vi "Configure Channel Probe.vi"(6 "Probe Signal Type (1: Single-ended)":i32(ring)=1 items=["Differential", "Single-ended"], 7 "Skew Factor (1E-7 S)":dbl=1e-07, 8 "error in (no error)":errorcluster, 9 "Probe Head Type (8: NONE)":i32(ring)=8 items=["Single- ended, 0dB", "Single- ended, 6dB", "Single- ended, 12dB", "Single- ended, 20dB", "Differential, 0dB", "Differential, 6dB", "Differential, 12dB", "Differential, 20dB", "NONE"], 10 "Channel Name (0: Channel 1)":i32(ring) items=["Channel 1", "Channel 2", "Channel 3", "Channel 4"], 11 "VISA resource name":refnum<visa-resource-name>) -> (0 "error out":errorcluster, 3 "VISA resource name out":refnum<visa-resource-name>)   [LabVIEW 2010, in "Agilent 2000 3000 X-Series.lvlib"]
doc: "Configures the channel probe."
uses:
  <instrlib>/Agilent 2000 3000 X-Series/Agilent 2000 3000 X-Series.lvlib
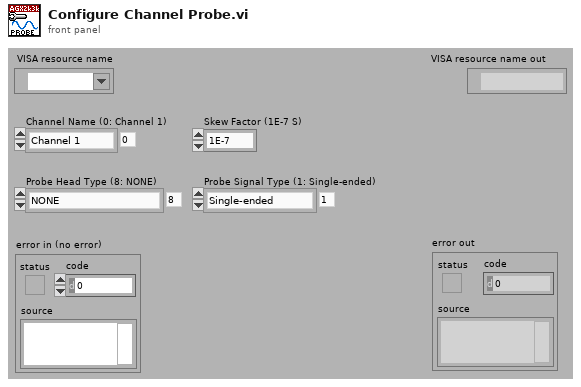
[diagram p1: front panel]
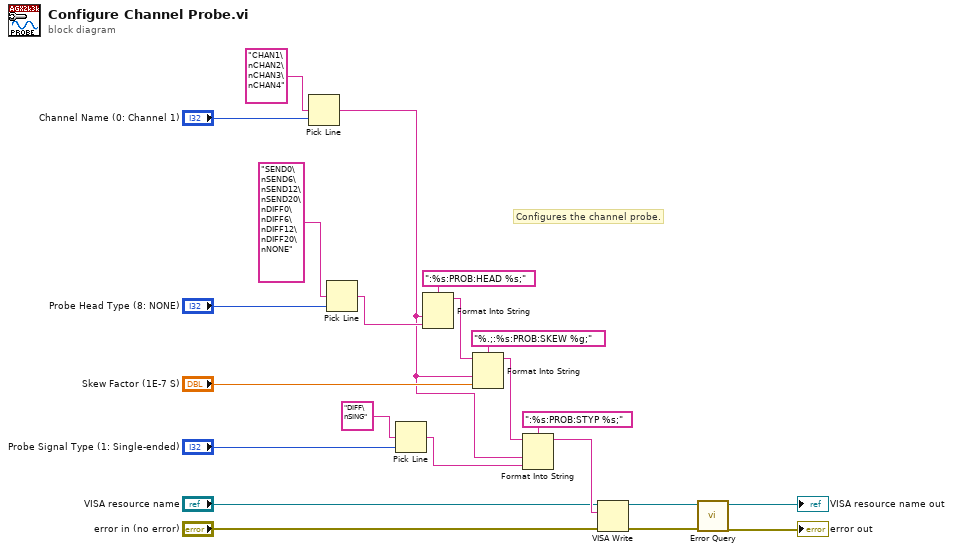
[diagram p0: block diagram]
diagram:
  # "Configures the channel probe."
  n1 = Pick Line(multi-line string="CHAN1\nCHAN2\nCHAN3\nCHAN4", line index="Channel Name (0: Channel 1)") -> (output string=w1:string)  [unwired: 1 out]
  n2 = Pick Line(multi-line string="SEND0\nSEND6\nSEND12\nSEND20\nDIFF0\nDIFF6\nDIFF12\nDIFF20\nNONE", line index="Probe Head Type (8: NONE)") -> (output string=w19:string)  [unwired: 1 out]
  n3 = Pick Line(multi-line string="DIFF\nSING", line index="Probe Signal Type (1: Single-ended)") -> (output string=w11:string)  [unwired: 1 out]
  n4 = Format Into String(format string=":%s:PROB:HEAD %s;", w1, w19) -> (resulting string=w18:string)  [unwired: 2 in, 1 out]
  n5 = Format Into String(format string="%.;:%s:PROB:SKEW %g;", initial string=w18, w1, "Skew Factor (1E-7 S)") -> (resulting string=w13:string)  [unwired: 1 in, 1 out]
  n6 = Format Into String(format string=":%s:PROB:STYP %s;", initial string=w13, w1, w11) -> (resulting string=w10:string)  [unwired: 1 in, 1 out]
  n7 = VISA Write(VISA resource name="VISA resource name", write buffer=w10, error in (no error)="error in (no error)") -> (VISA resource name out=w7:refnum<visa-resource-name>, error out=w6:errorcluster)  [unwired: 1 out]
  n8 = call <instrlib>:"Error Query.vi"("error in (no error)"=w6, "VISA resource name"=w7) -> ("error out"=→"error out":errorcluster, "VISA resource name out"=→"VISA resource name out":refnum<visa-resource-name>)  [unwired: 8 out]
